vi "CLD 2 Elapsed Time Express FGV Exercise.vi"(7 "Express Timer FGV Enum":enum16{"Reset", "Read Status", "Set Auto Reset"}(ring), 8 "error in (no error)":errorcluster, 9 "Auto Reset (F)":bool, 11 "Time Target (s)":dbl=7.0) -> (0 "error out":errorcluster, 2 "Elapsed Time (s)":dbl, 3 "Time Has Elapsed":bool)   [LabVIEW 2021]
doc: "CLD 2 Exercise"
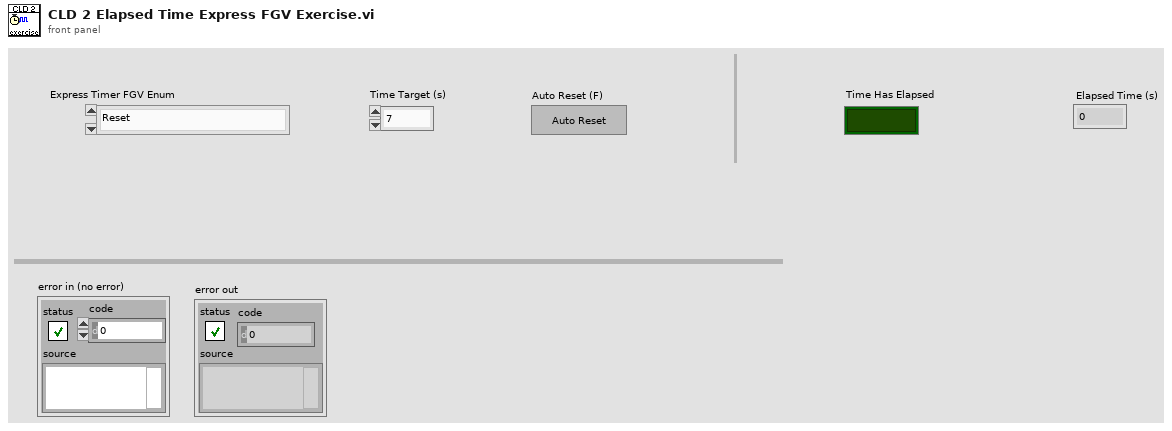
[diagram p1: front panel]
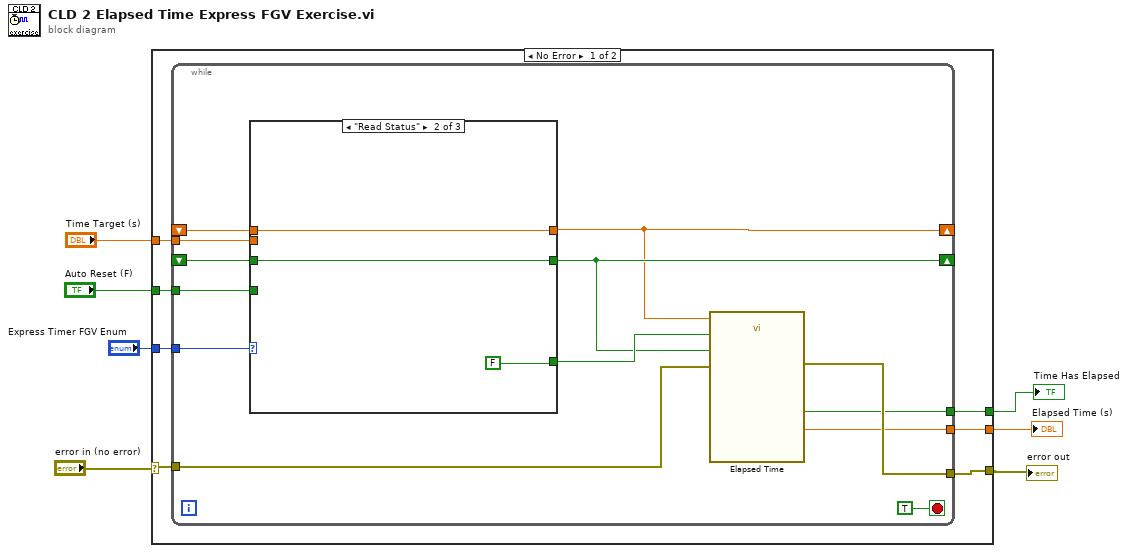
[diagram p0: block diagram]
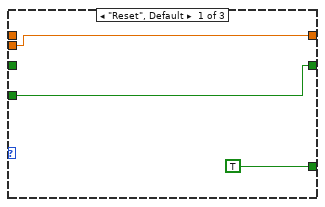
[diagram p2: hidden frame]
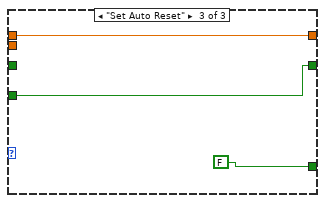
[diagram p3: hidden frame]
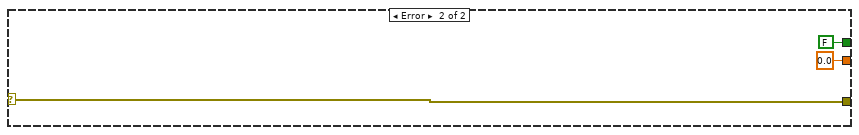
[diagram p4: hidden frame]
diagram:
  n1 = case shown="No Error" "error in (no error)" {
    selector: "error in (no error)" -> [w13 w39]
    tunnel: "Express Timer FGV Enum" -> [w14 _]
    tunnel: [w12 w39] -> w5
    tunnel: [w11 0.0 ("Elapsed Time (s)")] -> w4
    tunnel: [w10 FALSE ("Time has Elapsed")] -> w3
    tunnel: "Auto Reset (F)" -> [w9 _]
    tunnel: "Time Target (s)" -> [w8 _]
    frame No Error {
      n2 = while {
        tunnel: w14 -> [w27]
        tunnel: w13 -> [w26]
        tunnel: [w25] -> w12
        tunnel: [w24] -> w11
        tunnel: [w23] -> w10
        shift-right: [w17] -> _
        shift-left: _ -> [w22]
        tunnel: w9 -> [w21]
        tunnel: w8 -> [w19]
        shift-right: [w16] -> _
        shift-left: _ -> [w18]
        stop <- TRUE stop-if-true
        n3 = case shown="\"Read Status\"" w27 {
          tunnel: [w28 w33 w36] -> w17
          tunnel: w22 -> [_ w33 _]
          tunnel: w21 -> [w28 _ w36]
          tunnel: [TRUE FALSE FALSE] -> w20
          tunnel: w19 -> [w29 _ _]
          tunnel: [w29 w32 w35] -> w16
          tunnel: w18 -> [_ w32 w35]
          frame "Reset", Default {
          }
          frame "Read Status" {
          }
          frame "Set Auto Reset" {
          }
        }
        n4 = call "Elapsed Time"("Time Target (s)"=w16, "Reset"=w20, "Auto Reset"=w17, "error in (no error)"=w26) -> ("Elapsed Time (s)"=w24:dbl, "Time has Elapsed"=w23:bool, "error out"=w25:errorcluster)  [unwired: 8 in, 5 out]
      }
    }
    frame Error {
    }
  }
  "error out" <- w5
  "Elapsed Time (s)" <- w4
  "Time Has Elapsed" <- w3
